vi "Data Viewer.vi"() -> ()   [LabVIEW 2018]
uses:
  Type Defs/State Machine.ctl
  R-D-Developments/Type/_Data.ctl
  Function Lib.lvlib
  Type Defs/Data Viewer.ctl
panel:
  out "Error Out":errorcluster
  in  "Error In":errorcluster
  in  "MR#":i32=1 caption="MR #"
  in  "Expt#":i32=1 caption="Expt #"
  in  "Scan#":i32=1 caption="Scan #"
  in  "Avg":bool
  in  "Log":bool
  in  "CPS":bool
  out "Spectrum":cluster{"X":sgl[], "Y":sgl[]}(graph) caption="C:\\Users\\ ... /41. Stability-PPG(+)-20ulmin-90NG-5500-50 Cycles.isd; TIC=1114041; T=0mS"
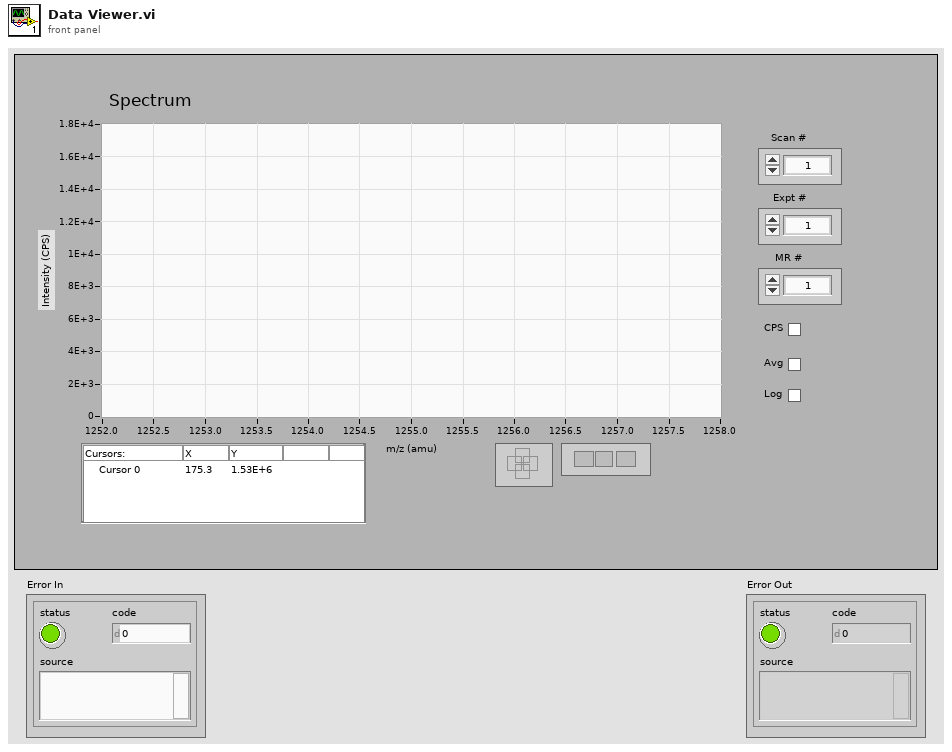
[diagram p1: front panel]
types:
  T1 = typedef "Data Viewer.ctl" = cluster{"Spectrum Data":T2, "Spectrum":refnum<vi>, "TIC VS Time":refnum<vi>, "Path":path, "TIC Spectrum":refnum<vi>, "TIC VS Time Offset":dbl, "Overlay Offset":dbl, "XIC Data":T2, "Offset":dbl, "File Offset":dbl[], "Overlay Data":cluster{"X":sgl[], "Y":sgl[]}[], "TIC Spectrum":T2}
  T2 = typedef "Function Lib.lvlib/_Data.ctl" = cluster{"X":dbl[], "Y":dbl[], "Dwell Time (mS)":dbl, "X Title":string, "Time (s)":dbl, "TIC":u32, "# of Scans":i32, "Path":path, "ScanType":i32}
  T3 = typedef "State Machine.ctl" = enum16{"Wait", "Init", "Case 0", "Case 1", "Case 2", "Case 3", "Case 4", "Case 5", "Case 6", "Case 7", "Case 8", "Case 9", "Case 10", "Error", "Exit"}
  T4 = enum32{"existing file", "new file", "new or existing file", "existing dir", "new dir", "new or existing dir", "existing file (use LLBs)", "new file (use LLBs)", "new or existing file (use LLBs)", "new or existing file or directory (use LLBs)"}
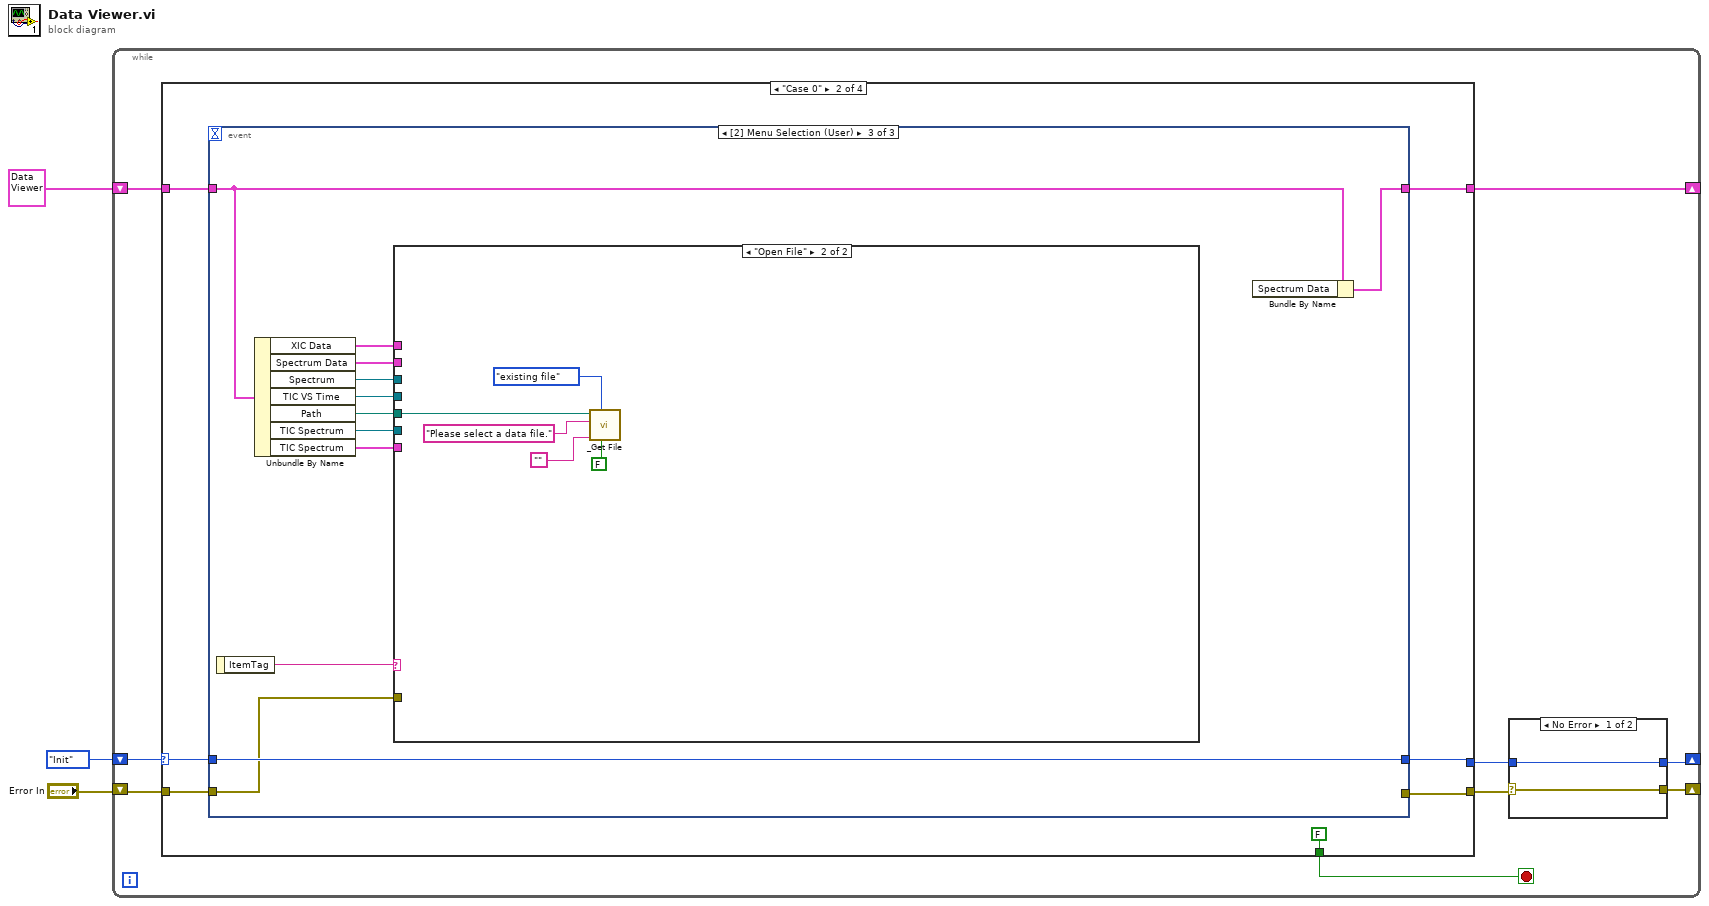
[diagram p0: block diagram]
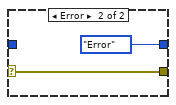
[diagram p2: hidden frame]
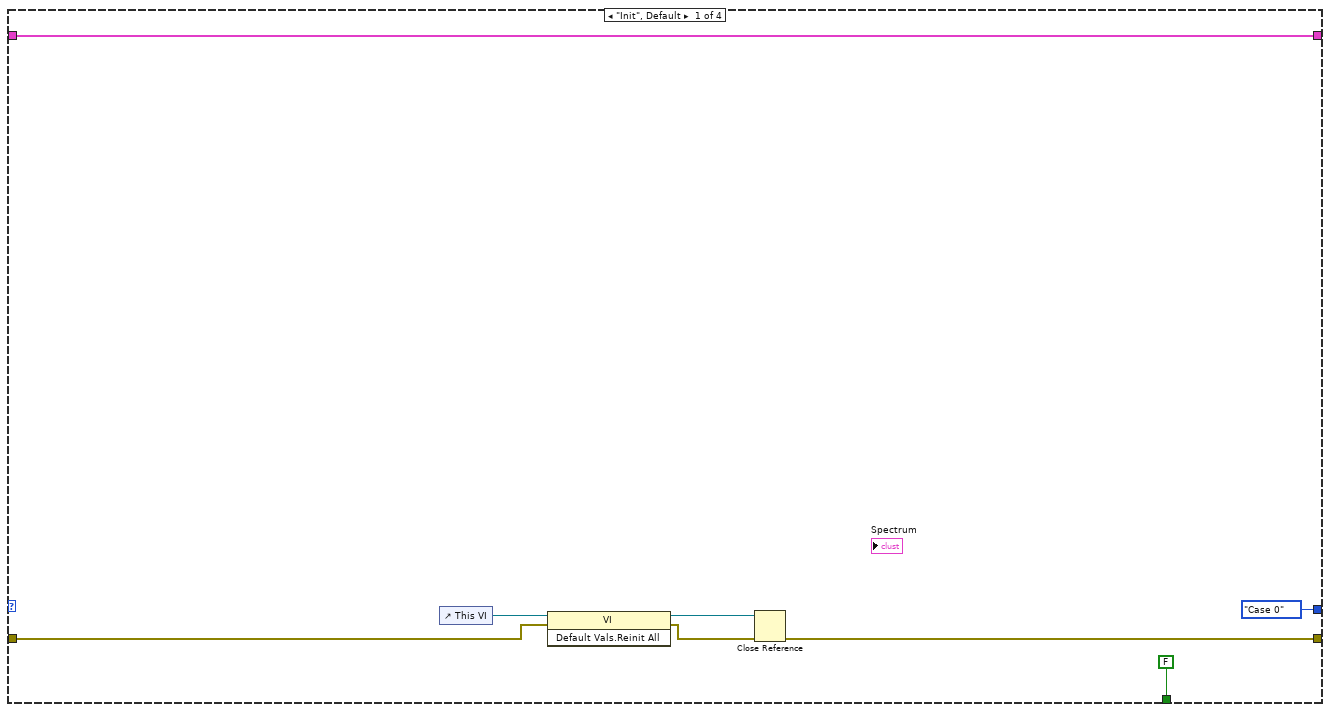
[diagram p3: hidden frame]
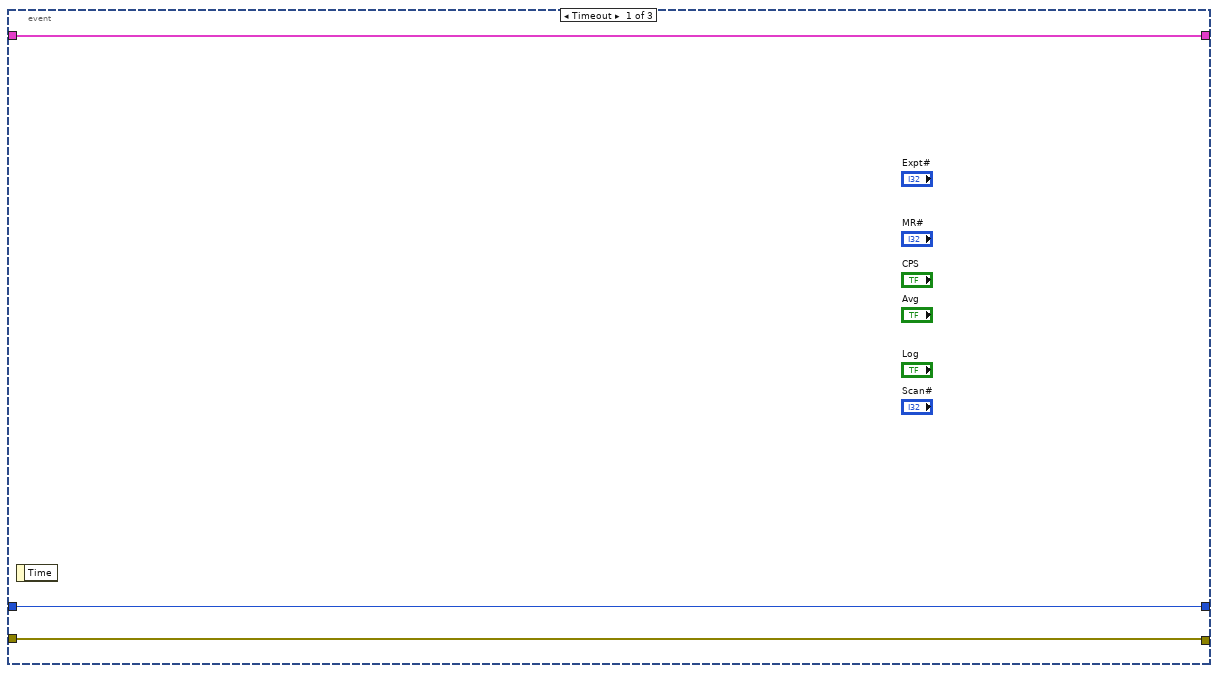
[diagram p4: hidden frame]
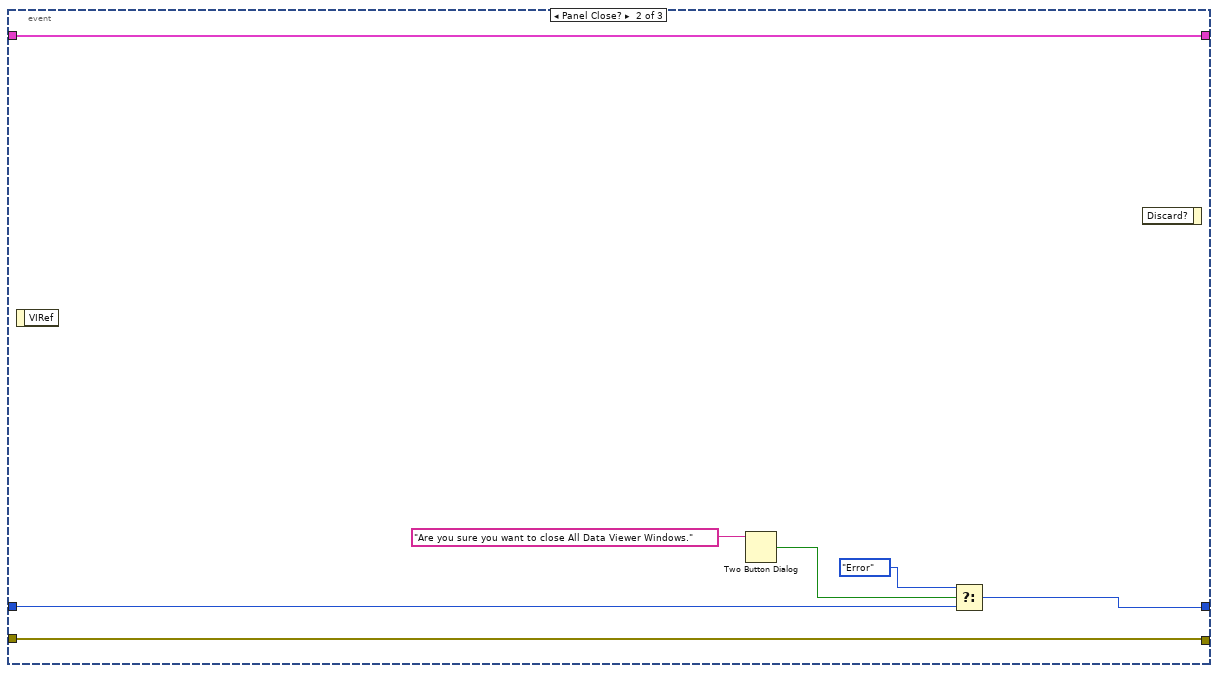
[diagram p5: hidden frame]
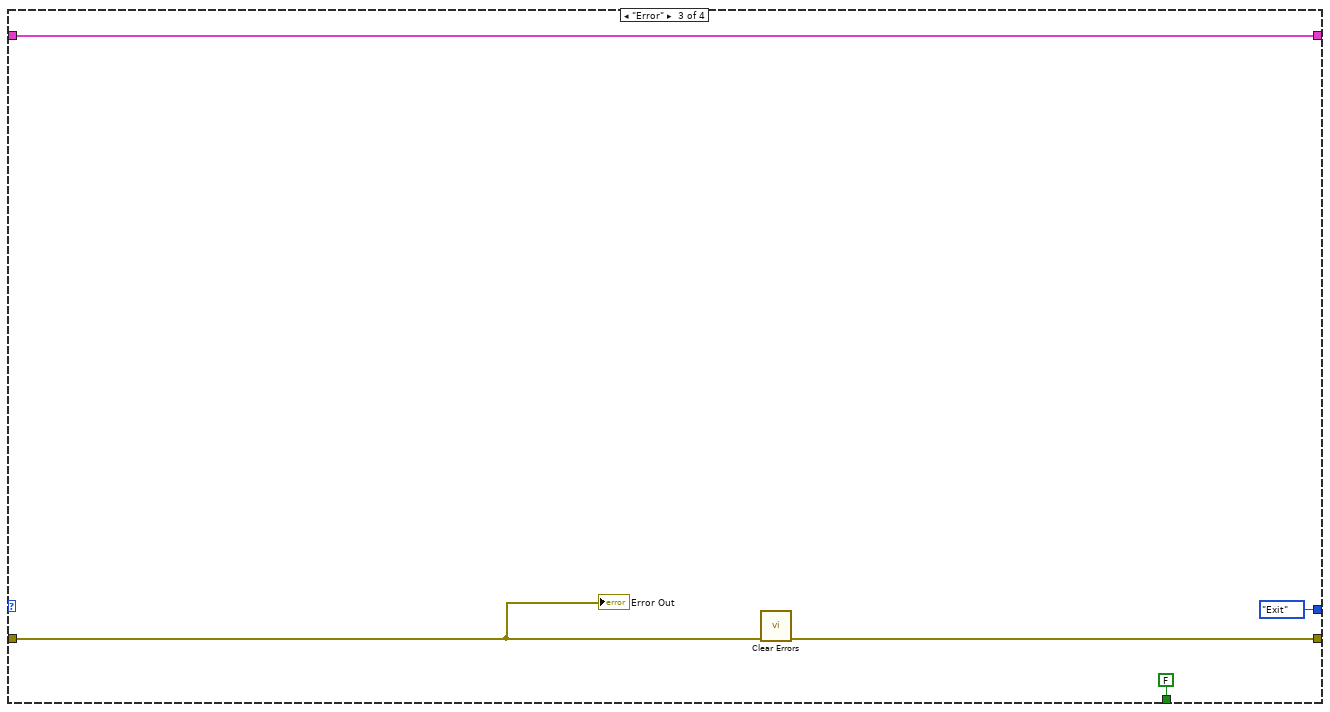
[diagram p7: hidden frame]
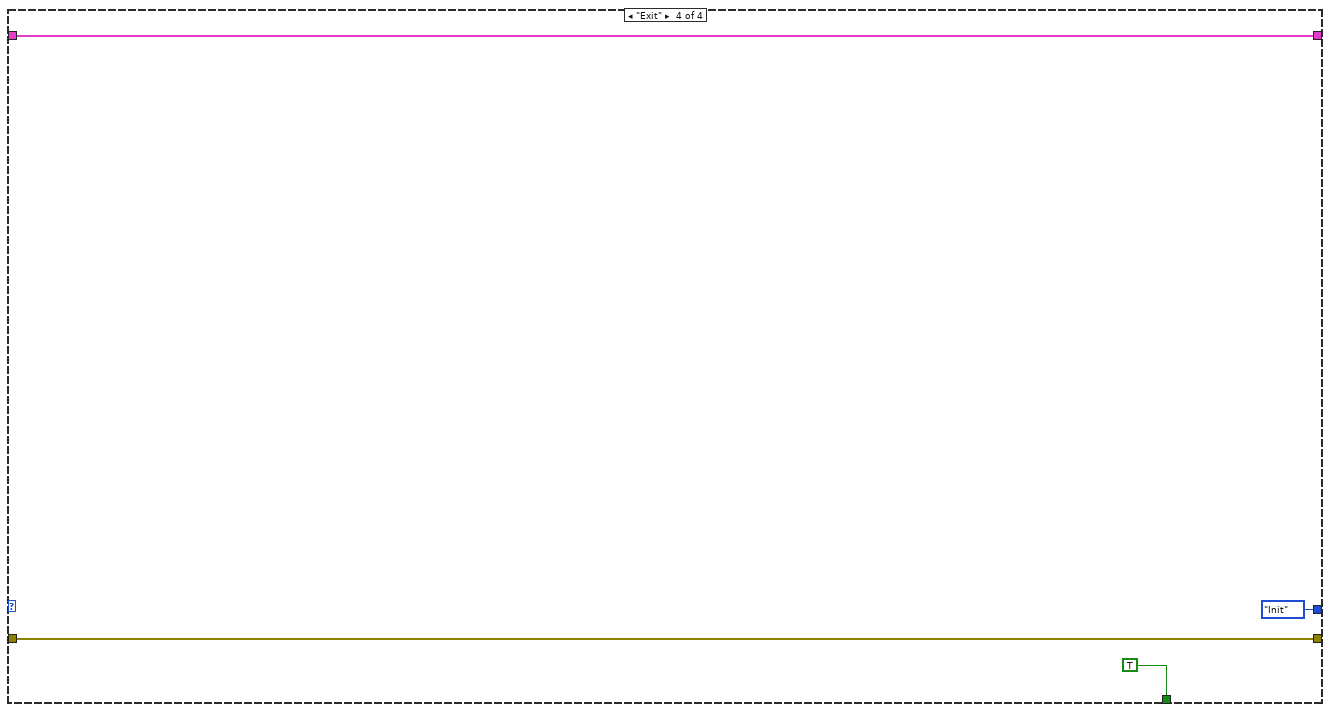
[diagram p8: hidden frame]
diagram:
  n1 = while {
    shift-right: [w9] -> _
    shift-left: State_Machine."Init" ("Enum") -> [w12]
    shift-right: [w7] -> _
    shift-left: "Error In" -> [w11]
    shift-right: [w4] -> _
    shift-left: T1 {"Spectrum Data"={"X"=[], "Y"=[], "Dwell Time (mS)"=0.0, "X Title"="", "Time (s)"=0.0, "TIC"=0, "# of Scans"=0, "Path"=path "", "ScanType"=0}, "Spectrum"=refnum, "TIC VS Time"=refnum, "Path"=path "", "TIC Spectrum"=refnum, "TIC VS Time Offset"=0.0, "Overlay Offset"=0.0, "XIC Data"={"X"=[], "Y"=[], "Dwell Time (mS)"=10.0, "X Title"="", "Time (s)"=0.0, "TIC"=0, "# of Scans"=133, "Path"=path "", "ScanType"=1}, "Offset"=0.0, "File Offset"=[], "Overlay Data"=[], "TIC Spectrum"={"X"=[], "Y"=[], "Dwell Time (mS)"=10.0, "X Title"="", "Time (s)"=0.0, "TIC"=0, "# of Scans"=133, "Path"=path "", "ScanType"=1}} ("Cluster") -> [w5]
    stop <- w6 stop-if-true
    n2 = case shown="\"Case 0\"" w12 {
      selector: w12 -> [_ w28 _ _]
      tunnel: w11 -> [w20 w30 w61 w66]
      tunnel: [w17 w29 w60 w66] -> w10
      tunnel: [State_Machine."Case 0" ("Enum") w27 State_Machine."Exit" ("Enum") State_Machine."Init" ("Enum")] -> w8
      tunnel: [FALSE FALSE FALSE TRUE] -> w6
      tunnel: w5 -> [w22 w26 w59 w64]
      tunnel: [w22 w25 w59 w64] -> w4
      frame "Init", Default {
        n3 = control-ref of="This VI"() -> (w21:refnum<vi>)
        n4 = invoke class="VI" method="Default Vals.Reinit All"(reference=w21, error in=w20) -> (reference out=w19:refnum<vi>, error out=w18:errorcluster)  [unwired: 1 in, 1 out]
        n5 = Close Reference(reference=w19, error in (no error)=w18) -> (error out=w17:errorcluster)
      }
      frame "Case 0" {
        n6 = event shown="[2] Menu Selection (User)" {
          selector: _ -> [_ _ _]
          dyn-events: _ -> [_ _ _]
          timeout: _ -> [_ _ _]
          tunnel: [w34 w41 _] -> w29
          tunnel: w30 -> [w34 w41 w51]
          tunnel: w28 -> [w33 w38 w52]
          tunnel: [w33 w37 w52] -> w27
          tunnel: w26 -> [w32 w35 w49]
          tunnel: [w32 w35 w50] -> w25
          event Timeout {
            n7 = event-data() -> ()  [unwired: 1 in, 1 out]
          }
          event Panel Close? {
            n8 = event-data() -> ()  [unwired: 1 in, 1 out]
            n9 = Two Button Dialog(message="Are you sure you want to close All Data Viewer Windows.") -> (T button?=w39:bool)  [unwired: 2 out]
            n10 = Select(t=State_Machine."Error" ("Enum"), s=w39, f=w38) -> (s? t:f=w37:T3)
            n11 = event-data() -> ()  [unwired: 2 in, 1 out]
          }
          event Menu Selection (User) {
            n12 = event-data() -> ("ItemTag"=w53:string)  [unwired: 1 in]
            n13 = Unbundle By Name(w49) -> ("XIC Data"=w48:T2, "Spectrum Data"=w47:T2, "Spectrum"=w46:refnum<vi>, "TIC VS Time"=w45:refnum<vi>, "Path"=w44:path, "TIC Spectrum"=w43:refnum<vi>, "TIC Spectrum"=w42:T2)
            n14 = case shown="\"Open File\"" w53 {
              tunnel: w51 -> [_ _]
              tunnel: w48 -> [_ _]
              tunnel: w47 -> [_ _]
              tunnel: w46 -> [_ _]
              tunnel: w45 -> [_ _]
              tunnel: w44 -> [_ w58]
              tunnel: w43 -> [_ _]
              tunnel: w42 -> [_ _]
              frame "False", Default {
              }
              frame "Open File" {
                n15 = call "_Get File.vi"("For Write (T)"=FALSE, "select mode (new or existing)"=T4."existing file", "default name"="", "prompt"="Please select a data file.", "Start Path"=w58) -> ()  [unwired: 1 in, 4 out]
              }
            }
            n16 = Bundle By Name(cluster=w49) -> (w50:T1)  [unwired: 1 in]
          }
        }
      }
      frame "Error" {
        n17 = call <vilib>:"Clear Errors.vi"("error in (no error)"=w61) -> ("error out"=w60:errorcluster)  [unwired: 5 in, 1 out]
        "Error Out" <- w61
      }
      frame "Exit" {
      }
    }
    n18 = case shown="No Error" w10 {
      selector: w10 -> [w13 w15]
      tunnel: [w14 State_Machine."Error" ("Enum")] -> w9
      tunnel: w8 -> [w14 _]
      tunnel: [w13 w15] -> w7
      frame No Error {
      }
      frame Error {
      }
    }
  }
